vi "FPGA Read Front Sonar.vi"(1 "stop":bool) -> (0 "Time of Flight":u32)   [LabVIEW 2015]
uses:
  <vilib>/rvi/Emulation/niFpgaGetClockAttributes.vi
  <vilib>/rvi/Emulation/niFpgaSctlEmulationGetInTimedLoop.vi
  <vilib>/rvi/Emulation/niFpgaEmulationReportErrorSimple.vi
  <vilib>/rvi/eio/common/nirviEmuTemplateMethod_errors.vi
  <vilib>/rvi/Emulation/niFpgaCriticalErrorInLSC.vi
  <vilib>/rvi/Emulation/niFpgaProcessEmulError.vi
  <vilib>/eio/EIONode/EIONode.xnode
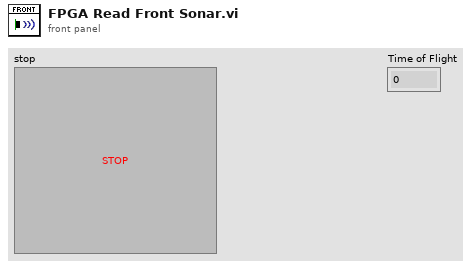
[diagram p1: front panel]
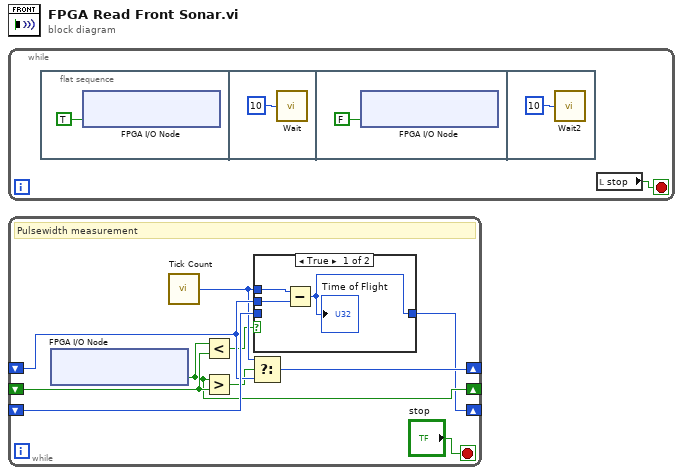
[diagram p0: block diagram]
diagram:
  n1 = while {
    stop <- w1 stop-if-true
    n2 = flat-sequence {
      frame #0 {
        n3 = xnode "FPGA I/O Node"("ConnectorB/DIO4"=TRUE) -> ()  [unwired: 1 in, 1 out]
      }
      frame #1 {
        n4 = call "Wait"("Count(uSec)"=u32 10 ("Count(mSec)")) -> ()  [unwired: 1 out]
      }
      frame #2 {
        n5 = xnode "FPGA I/O Node"("ConnectorB/DIO4"=FALSE) -> ()  [unwired: 1 in, 1 out]
      }
      frame #3 {
        n6 = call "Wait2"("Count(mSec)"=u32 10) -> ()  [unwired: 1 out]
      }
    }
    n7 = local read "stop"() -> (w1:bool)
  }
  n8 = while "Pulsewidth Measurement + Sound Output" {
    shift-left: _ -> [w15]
    shift-right: [w7] -> _
    shift-left: _ -> [w14]
    shift-right: [w13] -> _
    shift-left: _ -> [w11]
    shift-right: [w8] -> _
    stop <- "stop" stop-if-true
    # "Pulsewidth measurement"
    n9 = xnode "FPGA I/O Node"() -> ("ConnectorB/DIO7"=w8:bool)  [unwired: 1 in, 1 out]
    n10 = call "Tick Count"() -> ("Tick Count(uSec)"=w10:u32)
    n11 = Less?(x=w8, y=w11) -> (x < y?=w9:bool)
    n12 = Greater?(x=w8, y=w11) -> (0:w12:bool)
    n13 = Select(t=w10, s=w12, f=w14) -> (s? t:f=w13:u32)
    n14 = case shown="True" w9 {
      tunnel: w15 -> [_ w19]
      tunnel: w10 -> [w17 _]
      tunnel: w14 -> [w18 _]
      tunnel: [w16 w19] -> w7
      frame True {
        n15 = Subtract(x=w17, y=w18) -> (x-y=w16:u32)
        "Time of Flight" <- w16
      }
      frame False {
      }
    }
  }
